vi "GetSetControllerOptions.vi"(8 "error in":errorcluster, 9 "Option (may be added for multiple)":T1=8 items=["Product temperature control"=1, "Humidity system"=2, "Low humidity system"=4, "GSoak"=8, "Purge"=16, "Cascade refrigeration"=32, "Power Save mode"=64, "Single-stage refrig."=128, "Altitude"=512, "Mechanical boost"=1024, "Product dewpoint control"=32768], 10 "get/set":T2, 11 "VISA resource name":refnum<visa-resource-name>) -> (0 "error out":errorcluster, 2 "Option response":string, 3 "VISA resource name out":refnum<visa-resource-name>)   [LabVIEW 2023, in "Thermotron 8800.lvlib"]
doc: "OPTN\nCommand name: Send or load controller options\nCommand type: Variable\nDescription: The query command reads the options register of the 8800. If the 8800 is in manual mode, the operation command temporarily changes the 8800 options register to the new set of options. NOTE: If the selected options are not available on your chamber, the 8800 will return an error code.\nSyntax: OPTN? or OPTN[,]ddddd\nWhere ddddd is a coded integer up to five digits long, where each option has the following weight:\n1 Product temperature control \n2 Humidity system \n4 Low humidity system (SE-series only) \n8 GSoak \n16 Purge \n32 Cascade refrigeration (SE-series only) \n64 Power Save mode (SE-series only) \n128 Single-stage refrig. (SE-series only) \n256 Reserved (do not use) \n512 Altitude \n1024 Mechanical boost \n2048 Reserved (do not use) \n4096 Reserved (do not use) \n8192 Reserved (do not use) \n16384 Reserved (do not use) \n32768 Product dewpoint control\nThe code provides a value between 0 and 65535 that is the sum of the values of all the enabled options. For example, a value of 49 (49 = 32 + 16 + 1) indicates that the cascade refrigeration system (32), purge (16), and product temperature control (1) options are enabled.\nData type: Coded integer; see Syntax.\nQuery example: OPTN?\n8800 response: 130 (The single-stage refrigeration and humidity options are enabled.)\nOperation example: OPTN82\n8800 response: 0 (This command sets the 8800 manual mode options to enable Power Save, purge, and humidity.)"
uses:
  Thermotron 8800.lvlib
  Private/get set.ctl
  Private/OptionWordSelection.ctl
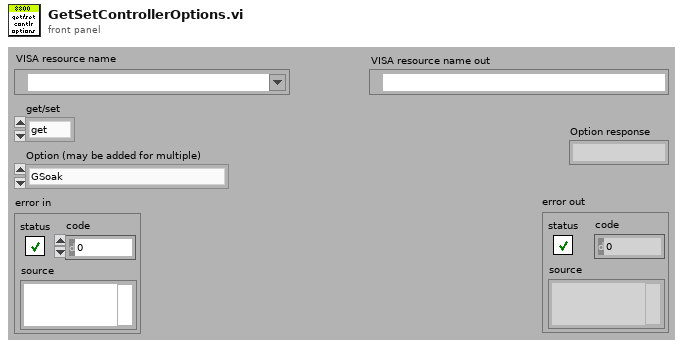
[diagram p1: front panel]
types:
  T1 = typedef "Thermotron 8800.lvlib/OptionWordSelection.ctl" = u16
  T2 = typedef "Thermotron 8800.lvlib/get set.ctl" = enum16{"get", "set"}
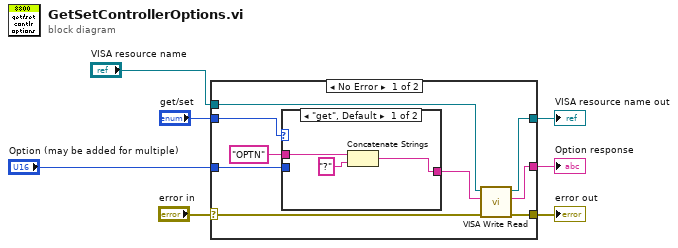
[diagram p0: block diagram]
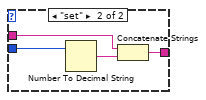
[diagram p2: hidden frame]
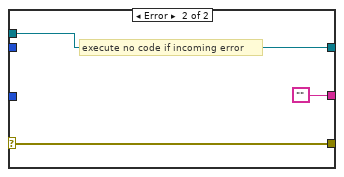
[diagram p3: hidden frame]
diagram:
  n1 = case shown="No Error" "error in" {
    selector: "error in" -> [w8 w25]
    tunnel: "get/set" -> [w16 _]
    tunnel: [w13 ""] -> w2
    tunnel: [w12 w25] -> w5
    tunnel: [w11 w26] -> w4
    tunnel: "VISA resource name" -> [w10 w26]
    tunnel: "Option (may be added for multiple)" -> [w9 _]
    frame No Error {
      n2 = case shown="\"get\", Default" w16 {
        tunnel: "OPTN" ("8800 Command") -> [w18 w23]
        tunnel: [w19 w22] -> w14
        tunnel: w9 -> [_ w20]
        frame "get", Default {
          n3 = Concatenate Strings(w18, "?" ("8800 Command")) -> (w19:string)
        }
        frame "set" {
          n4 = Number To Decimal String(number=w20) -> (decimal integer string=w21:string)  [unwired: 1 in]
          n5 = Concatenate Strings(w23, w21) -> (w22:string)
        }
      }
      n6 = call "VISA Write Read.vi"("error in (no error)"=w8, "8800 Command"=w14, "VISA Refnum in"=w10) -> ("error out"=w12:errorcluster, "read buffer"=w13:string, "VISA Refnum out"=w11:refnum<visa-resource-name>)  [unwired: 6 in]
    }
    frame Error {
      # "execute no code if incoming error"
    }
  }
  "VISA resource name out" <- w4
  "error out" <- w5
  "Option response" <- w2
